vi "Parse Response JSON.vi"(8 "error in (no error)":errorcluster, 10 "Response JSON":string, 11 "RGetStreamStatus in":refnum<class "RGetStreamStatus.lvclass">) -> (0 "error out":errorcluster, 3 "RGetStreamStatus out":refnum<class "RGetStreamStatus.lvclass">)   [LabVIEW 2020, in "obs-websocket.lvlib" / "RGetStreamStatus.lvclass"]
uses:
  RGetStreamStatus.lvclass
  Stream Status.ctl
  RGetStreamStatus.lvclass/RGetStreamStatus.ctl
  obs-websocket.lvlib
  <vilib>/JDP Science/JSONtext/JSONtext.lvlib
  74135cb5-5620-4d66-82eb-0e3f2193097b.vi
  c01915f8-ef3e-42e5-9760-0cc4e2e383f7.vi
  191b3109-aa90-4059-87d0-12b5d3f72e54.vi
  0562d6b0-09de-4a2d-b35a-3e7797ed2b5b.vi
  414553a5-7b1b-4cb2-b99e-b0595af342e6.vi
  f19cf33e-5418-40c7-b80e-39415fca1cbd.vi
  9920018b-5b58-467d-9f08-fd4bc2dcce07.vi
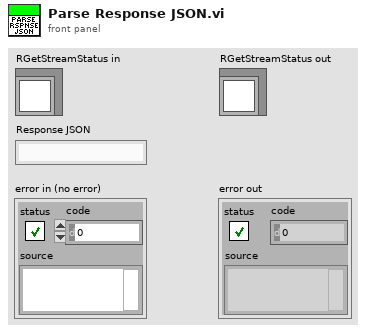
[diagram p1: front panel]
types:
  T1 = typedef "obs-websocket.lvlib/Stream Status.ctl" = cluster{"Active":bool, "Reconnecting":bool, "Timecode":string, "Duration mS":u32, "Bytes":u32, "Skipped Frames":u32, "Total Frames":u32}
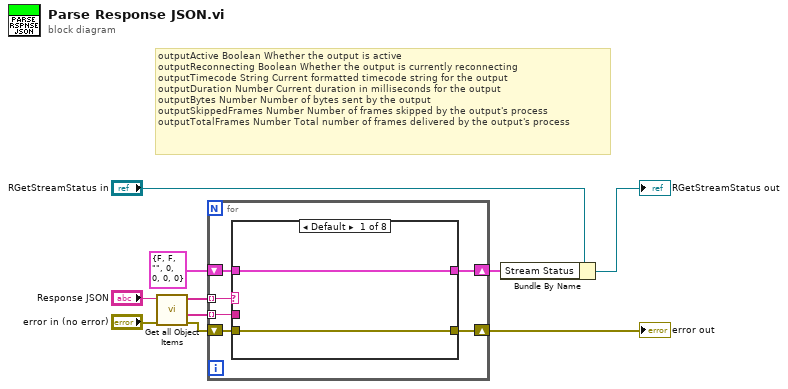
[diagram p0: block diagram]
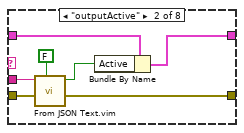
[diagram p2: hidden frame]
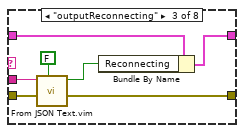
[diagram p3: hidden frame]
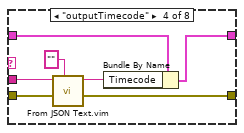
[diagram p4: hidden frame]
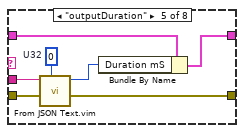
[diagram p5: hidden frame]
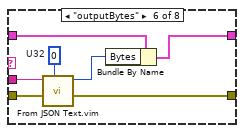
[diagram p6: hidden frame]
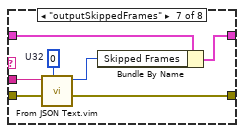
[diagram p7: hidden frame]
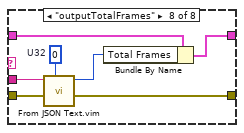
[diagram p8: hidden frame]
diagram:
  # "outputActive\tBoolean\tWhether the output is active\noutputReconnecting\tBoolean\tWhether the output is currently reconnecting\noutputTimecode\tString\tCurrent formatted timecode string for the output\noutputDuration\tNumber\tCurrent duration in milliseconds for the output\noutputBytes\tNumber\tNumber of bytes sent by the output\noutputSkippedFrames\tNumber\tNumber of frames skipped by the output's process\noutputTotalFrames\tNumber\tTotal number of frames delivered by the output's process"
  n1 = call <vilib>:"Get all Object Items.vi"("error in (no error)"="error in (no error)", "JSON"="Response JSON") -> ("error out"=w2:errorcluster, "<JSON>"=w3:string[], "Item Names"=w4:string[])  [unwired: 6 in, 1 out]
  n2 = for {
    tunnel: w3 -> [w15] mode=indexing
    tunnel: w4 -> [w16] mode=indexing
    shift-right: [w13] -> w6
    shift-left: T1 {"Active"=FALSE, "Reconnecting"=FALSE, "Timecode"="", "Duration mS"=0, "Bytes"=0, "Skipped Frames"=0, "Total Frames"=0} ("Stream Status") -> [w14]
    shift-right: [w12] -> w1
    shift-left: w2 -> [w11]
    n3 = case shown="Default" w16 {
      tunnel: w15 -> [_ w23 w30 w38 w44 w51 w58 w65]
      tunnel: w14 -> [w18 w25 w32 w39 w46 w53 w59 w66]
      tunnel: [w18 w24 w31 w37 w45 w52 w60 w67] -> w13
      tunnel: [w17 w19 w26 w34 w40 w47 w54 w61] -> w12
      tunnel: w11 -> [w17 w22 w29 w33 w43 w50 w57 w64]
      frame Default {
      }
      frame "outputActive" {
        n4 = call "From JSON Text.vim"("Data Type and Default Value"=FALSE, "error in (no error)"=w22, "JSON"=w23) -> ("error out"=w19:errorcluster, "Data out"=w20:bool)  [unwired: 7 in]
        n5 = Bundle By Name(cluster=w25, "Active"=w20) -> (w24:T1)
      }
      frame "outputReconnecting" {
        n6 = call "From JSON Text.vim"("Data Type and Default Value"=FALSE, "error in (no error)"=w29, "JSON"=w30) -> ("error out"=w26:errorcluster, "Data out"=w27:bool)  [unwired: 7 in]
        n7 = Bundle By Name(cluster=w32, "Reconnecting"=w27) -> (w31:T1)
      }
      frame "outputTimecode" {
        n8 = call "From JSON Text.vim"("Data Type and Default Value"="", "error in (no error)"=w33, "JSON"=w38) -> ("error out"=w34:errorcluster, "Data out"=w36:string)  [unwired: 7 in]
        n9 = Bundle By Name(cluster=w39, "Timecode"=w36) -> (w37:T1)
      }
      frame "outputDuration" {
        w42 = u32 0  # U32
        n10 = call "From JSON Text.vim"("Data Type and Default Value"=w42, "error in (no error)"=w43, "JSON"=w44) -> ("error out"=w40:errorcluster, "Data out"=w41:u32)  [unwired: 7 in]
        n11 = Bundle By Name(cluster=w46, "Duration mS"=w41) -> (w45:T1)
      }
      frame "outputBytes" {
        w49 = u32 0  # U32
        n12 = call "From JSON Text.vim"("Data Type and Default Value"=w49, "error in (no error)"=w50, "JSON"=w51) -> ("error out"=w47:errorcluster, "Data out"=w48:u32)  [unwired: 7 in]
        n13 = Bundle By Name(cluster=w53, "Bytes"=w48) -> (w52:T1)
      }
      frame "outputSkippedFrames" {
        w56 = u32 0  # U32
        n14 = call "From JSON Text.vim"("Data Type and Default Value"=w56, "error in (no error)"=w57, "JSON"=w58) -> ("error out"=w54:errorcluster, "Data out"=w55:u32)  [unwired: 7 in]
        n15 = Bundle By Name(cluster=w59, "Skipped Frames"=w55) -> (w60:T1)
      }
      frame "outputTotalFrames" {
        w63 = u32 0  # U32
        n16 = call "From JSON Text.vim"("Data Type and Default Value"=w63, "error in (no error)"=w64, "JSON"=w65) -> ("error out"=w61:errorcluster, "Data out"=w62:u32)  [unwired: 7 in]
        n17 = Bundle By Name(cluster=w66, "Total Frames"=w62) -> (w67:T1)
      }
    }
  }
  "error out" <- w1
  n18 = Bundle By Name(cluster="RGetStreamStatus in", "Stream Status"=w6) -> (→"RGetStreamStatus out":refnum<class "RGetStreamStatus.lvclass">)
